vi "AH2500_Set_Monitor_Values.vi"(5 "System Monitor Variables (in)":T1) -> (1 "System Monitor Variables (out)":T1)   [LabVIEW 2019]
uses:
  Global/Global Variables/System Monitor Cluster.ctl
  Global/Global Variables/Data_Display_global.vi
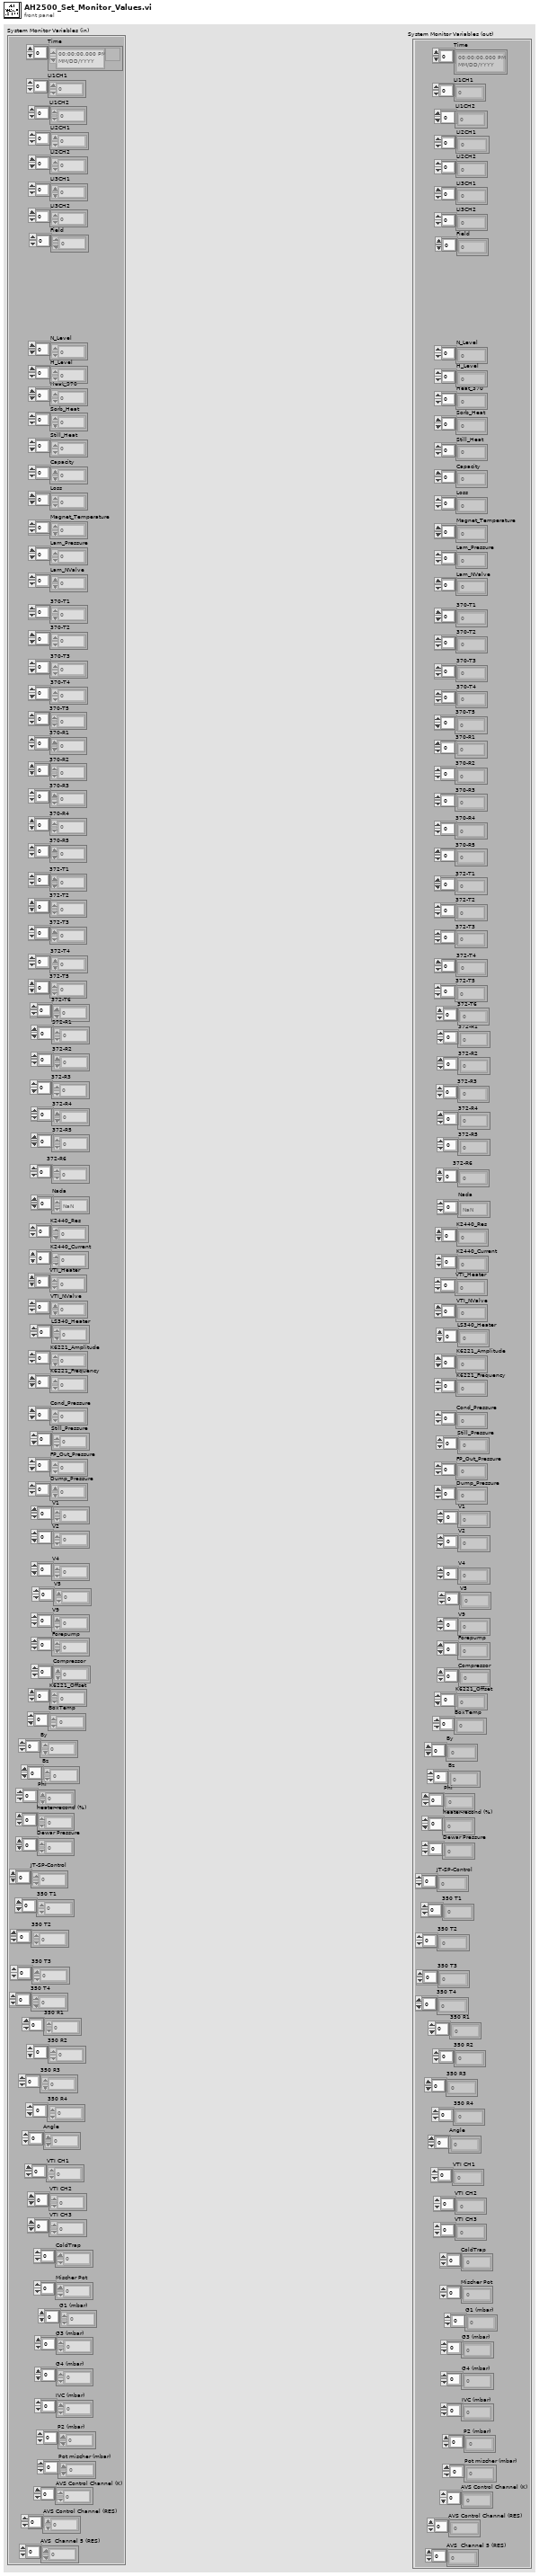
[diagram p1: front panel]
types:
  T1 = typedef "System Monitor Cluster.ctl" = cluster{"Time":timestamp[], "LI1CH1":dbl[], "LI1CH2":dbl[], "LI2CH1":dbl[], "LI2CH2":dbl[], "LI3CH1":dbl[], "LI3CH2":dbl[], "Field":dbl[], "N_Level":dbl[], "H_Level":dbl[], "Heat_370":dbl[], "Sorb_Heat":dbl[], "Still_Heat":dbl[], "Capacity":dbl[], "Loss":dbl[], "Magnet_Temperature":dbl[], "Lam_Pressure":dbl[], "Lam_NValve":dbl[], "370-T1":dbl[], "370-T2":dbl[], "370-T3":dbl[], "370-T4":dbl[], "370-T5":dbl[], "370-R1":dbl[], "370-R2":dbl[], "370-R3":dbl[], "370-R4":dbl[], "370-R5":dbl[], "372-T1":dbl[], "372-T2":dbl[], "372-T3":dbl[], "372-T4":dbl[], "372-T5":dbl[], "372-T6":dbl[], "372-R1":dbl[], "372-R2":dbl[], "372-R3":dbl[], "372-R4":dbl[], "372-R5":dbl[], "372-R6":dbl[], "Nada":dbl[], "K2440_Res":dbl[], "K2440_Current":dbl[], "VTI_Heater":dbl[], "VTI_NValve":dbl[], "LS340_Heater":dbl[], "K6221_Amplitude":dbl[], "K6221_Frequency":dbl[], "Cond_Pressure":dbl[], "Still_Pressure":dbl[], "FP_Out_Pressure":dbl[], "Dump_Pressure":dbl[], "V1":dbl[], "V2":dbl[], "V4":dbl[], "V5":dbl[], "V9":dbl[], "Forepump":dbl[], "Compressor":dbl[], "K6221_Offset":dbl[], "BoxTemp":dbl[], "By":dbl[], "Bz":dbl[], "Phi":dbl[], "heater-recond (%)":dbl[], "Dewar Pressure ":dbl[], "JT-SP-Control":dbl[], "350 T1":dbl[], "350 T2":dbl[], "350 T3":dbl[], "350 T4":dbl[], "350 R1":dbl[], "350 R2":dbl[], "350 R3":dbl[], "350 R4":dbl[], "Angle":dbl[], "VTI CH1":dbl[], "VTI CH2":dbl[], "VTI CH3":dbl[], "ColdTrap":dbl[], "Mischer Pot":dbl[], "G1 (mbar)":dbl[], "G3 (mbar) ":dbl[], "G4 (mbar)":dbl[], "IVC (mbar)":dbl[], "P2 (mbar) ":dbl[], "Pot mischer (mbar)":dbl[], "AVS Control Channel (K)":dbl[], "AVS Control Channel (RES)":dbl[], "AVS  Channel 5 (RES) ":dbl[]}
  T2 = typedef "AH2500-Cluster.ctl" = cluster{"Capacity Graphic":dbl[][], "Loss Graphic":dbl[][], "Update AH2500":bool, "Capacity":dbl, "Loss":dbl, "AVerage":enum16{"0", "1", "2", "3", "4", "5", "6", "7", "8", "9", "10", "11", "12", "13", "14", "15"}, "ALternate":enum16{"0", "1", "2", "3", "4", "5", "6", "7"}, "BIas":enum16{"Disabled", "100 MOhm", "1 MOhm"}, "V excitation":enum16{"15.00", "7.50", "3.75", "3.00", "1.50", "0.750", "0.375", "0.250", "0.125", "0.100", "0.050", "0.030", "0.015", "0.010", "0.0050", "0.0030", "0.0015", "0.0010", "0.0005"}}
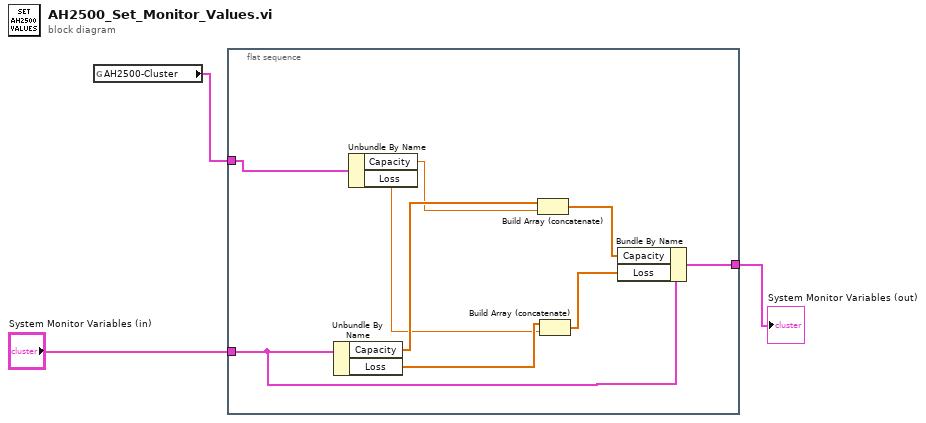
[diagram p0: block diagram]
diagram:
  n1 = global read "Data_Display_global.vi" "AH2500-Cluster"() -> (w3:T2)
  n2 = flat-sequence {
    tunnel: w3 -> [w12]
    tunnel: "System Monitor Variables (in)" -> [w7]
    tunnel: [w4] -> w1
    frame #0 {
      n3 = Unbundle By Name(w7) -> ("Capacity"=w11:dbl[], "Loss"=w9:dbl[])
      n4 = Unbundle By Name(w12) -> ("Capacity"=w10:dbl, "Loss"=w8:dbl)
      n5 = Build Array (concatenate)(w11, w10) -> (w6:dbl[])
      n6 = Build Array (concatenate)(w9, w8) -> (w5:dbl[])
      n7 = Bundle By Name(cluster=w7, "Capacity"=w6, "Loss"=w5) -> (w4:T1)
    }
  }
  "System Monitor Variables (out)" <- w1
